vi "mmWave Instrument Control Main.vi"   [LabVIEW 2019]
doc: "Main VI for instrument control"
uses:
  SubVIs/Shared/System GV.vi
  Modules/HW Control/HW Control.lvlib
  Modules/Log/Log.lvlib
  Modules/Data Managment/DataManagment.lvlib
  Modules/Communication Interface/Communication Interface.lvlib
  Modules/GUI/GUI.lvlib
  SubVIs/Shared/Shared.lvlib
  <vilib>/addons/_AddQ/G#Object/G#Object.lvclass
panel:
  # "mmWave Instrument Control\n-MAIN VI-"
types:
  T1 = enum32{"Invalid", "Standard", "Closed", "Hidden", "Minimized", "Maximized"}
  T2 = enum32{"invalid app kind", "Development System", "Run Time System", "Student Edition", "Embedded LabVIEW", "Evaluation", "Custom"}
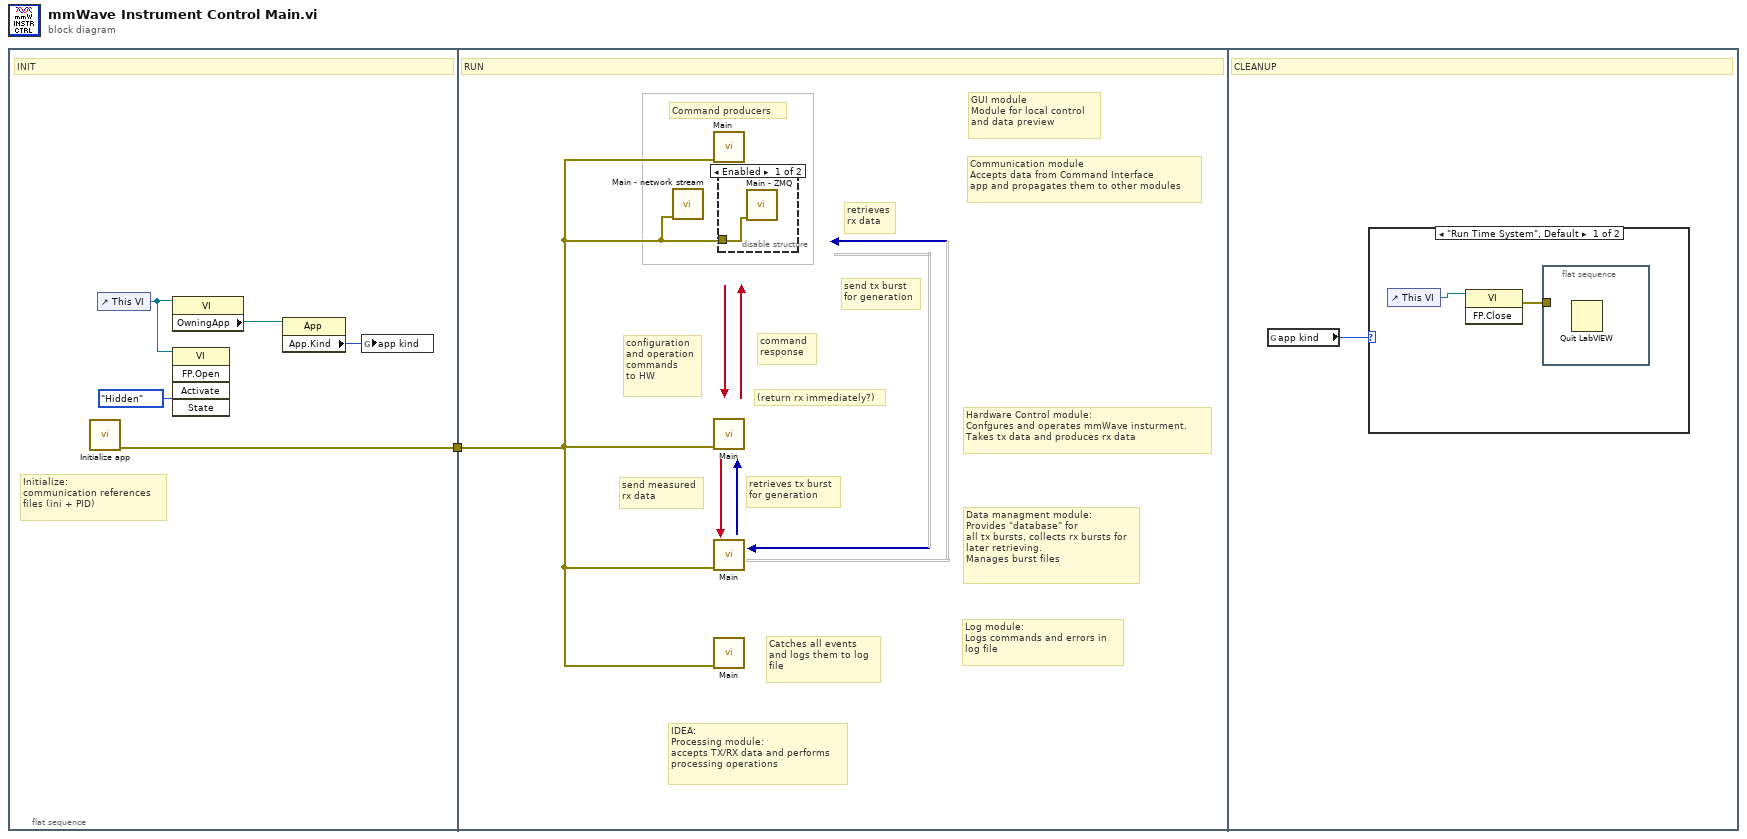
[diagram p0: block diagram]
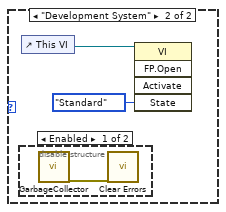
[diagram p3: hidden frame]
diagram:
  n1 = flat-sequence {
    tunnel: [w6] -> w1
    tunnel: w1 -> [w7]
    frame #0 {
      # "Initialize:\ncommunication references\nfiles (ini + PID)"
      # "INIT"
      n2 = call "Initialize app.vi"() -> ("error out"=w6:errorcluster)  [unwired: 11 in]
      n3 = control-ref of="This VI"() -> (w4:refnum<vi>)
      n4 = property class="VI"(reference=w4) -> ("OwningApp"=w3:refnum<vi>)  [unwired: 1 in, 2 out]
      n5 = invoke class="VI" method="FP.Open"(reference=w4, "State"=T1."Hidden") -> ()  [unwired: 3 in, 5 out]
      n6 = property class="App"(reference=w3) -> ("App.Kind"=w2:T2)  [unwired: 1 in, 2 out]
      n7 = global write "System GV.vi" "app kind"(w2) -> ()
    }
    frame #1 {
      # "Command producers"
      # "GUI module\nModule for local control\nand data preview"
      # "(return rx immediately?)"
      # "IDEA:\nProcessing module:\naccepts TX/RX data and performs\nprocessing operations"
      # "Log module:\nLogs commands and errors in\nlog file"
      # "Data managment module:\nProvides \"database\" for\nall tx bursts, collects rx bursts for\nlater retrieving.\nManages burst files"
      # "Hardware Control module:\nConfgures and operates mmWave insturment.\nTakes tx data and produces rx data"
      # "Communication module\nAccepts data from Command Interface\napp and propagates them to other modules"
      # "Catches all events\nand logs them to log\nfile"
      # "retrieves tx burst \nfor generation"
      # "send measured\nrx data"
      # "retrieves \nrx data"
      # "send tx burst \nfor generation"
      # "command\nresponse"
      # "configuration\nand operation\ncommands\nto HW"
      # "RUN"
      n8 = call "Main - network stream.vi"("error in (no error)"=w7) -> ()  [unwired: 10 in, 1 out]
      n9 = call "Main.vi"("error in (no error)"=w7) -> ()  [unwired: 10 in, 1 out]
      n10 = call "Main.vi"("error in (no error)"=w7) -> ()  [unwired: 10 in, 1 out]
      n11 = call "Main.vi"("error in (no error)"=w7) -> ()  [unwired: 10 in, 1 out]
      n12 = call "Main.vi"("error in (no error)"=w7) -> ()  [unwired: 10 in, 1 out]
      n13 = disable-structure shown="Enabled" {
        disable-tunnel: w7 -> [w8 _]
        frame Enabled {
          n14 = call "Main - ZMQ.vi"("error in (no error)"=w8) -> ()  [unwired: 10 in, 1 out]
        }
        frame Disabled {
        }
      }
    }
    frame #2 {
      # "CLEANUP"
      n15 = global read "System GV.vi" "app kind"() -> (w9:T2)
      n16 = case shown="\"Run Time System\", Default" w9 {
        frame "Run Time System", Default {
          n17 = control-ref of="This VI"() -> (w11:refnum<vi>)
          n18 = invoke class="VI" method="FP.Close"(reference=w11) -> (error out=w10:errorcluster)  [unwired: 2 in, 2 out]
          n19 = flat-sequence {
            tunnel: w10 -> [_]
            frame #0 {
              n20 = Quit LabVIEW() -> ()  [unwired: 1 in]
            }
          }
        }
        frame "Development System" {
          n21 = disable-structure shown="Enabled" {
            frame Enabled {
              n22 = call <vilib>:"GarbageCollector.vi"() -> ("error out"=w14:errorcluster)  [unwired: 17 in, 2 out]
              n23 = call <vilib>:"Clear Errors.vi"("error in (no error)"=w14) -> ()  [unwired: 5 in, 2 out]
            }
            frame Disabled {
            }
          }
          n24 = control-ref of="This VI"() -> (w13:refnum<vi>)
          n25 = invoke class="VI" method="FP.Open"(reference=w13, "State"=T1."Standard") -> ()  [unwired: 3 in, 5 out]
        }
      }
    }
  }
